vi "TEST Config.vi"() -> ()   [LabVIEW 2013, in "Carya Config.lvclass"]
doc: "Copyright 2018, Carya Automatisering, Wiebe Walstra."
uses:
  Carya Config.lvclass
  CConfig Object/Data.ctl
  CConfig Object/CConfig Object.lvclass
  CConfig Object/Set Query/Set Query.lvclass
  CConfig Object/Step In Query/Step In Query.lvclass
  CConfig Object/Loop Query/Match Query/Match Query.lvclass
  CConfig Object/Loop Query/All Query/All Query.lvclass
panel:
  out "Section names 5":string[](array[string])
  out "Array 2":string[](array[string])
  out "String 7":string
  out "String 6":string
  out "Section names 4":string[](array[string])
  out "Key names 3":string[](array[string])
  out "Key names 2":string[](array[string])
  out "Section names 3":string[](array[string])
  out "Section names 2":string[](array[string])
  out "String 5":string
  out "Key names":string[](array[string])
  out "Section names":string[](array[string])
  out "String 4":string
  out "Section names":string[](array[string])
  out "Key context":string[](array[string])
  out "Key names":string[](array[string])
  out "Section names":string[](array[string])
  out "Array":bool[][](array[boolean])
  out "String 3":string
  out "Found?":bool
  in  "String 2":string="[123]\none=test\na=aval\nb=bval\nc=cval\nd=dval\n13=abcval\n\n[456]\ntwo=abc\nstring=\"\"\nstring2=\"\""
  out "Value":string
  out "String":string
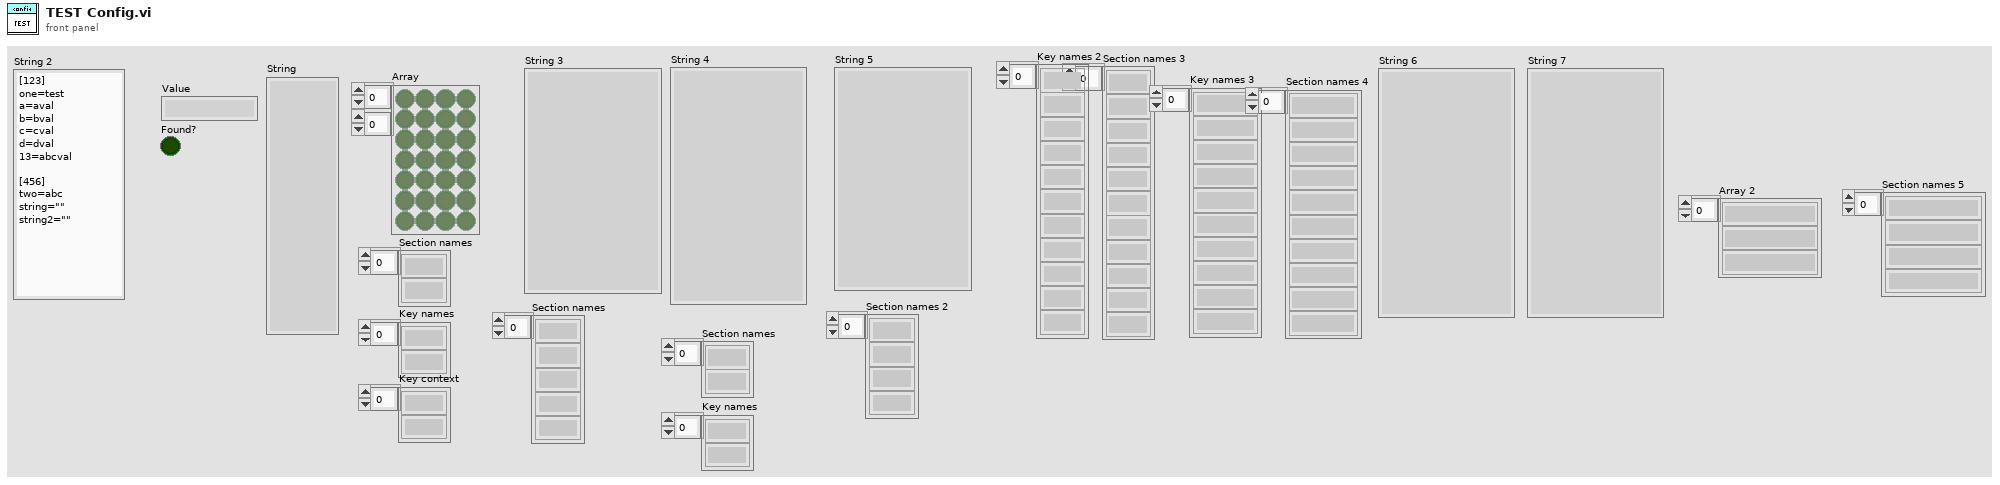
[diagram p1: front panel]
types:
  T1 = typedef "CConfig Object.lvclass/Data.ctl" = enum16{"pre", "name", "middle", "value", "post", "newline", "persistant", "tagged", "type"}
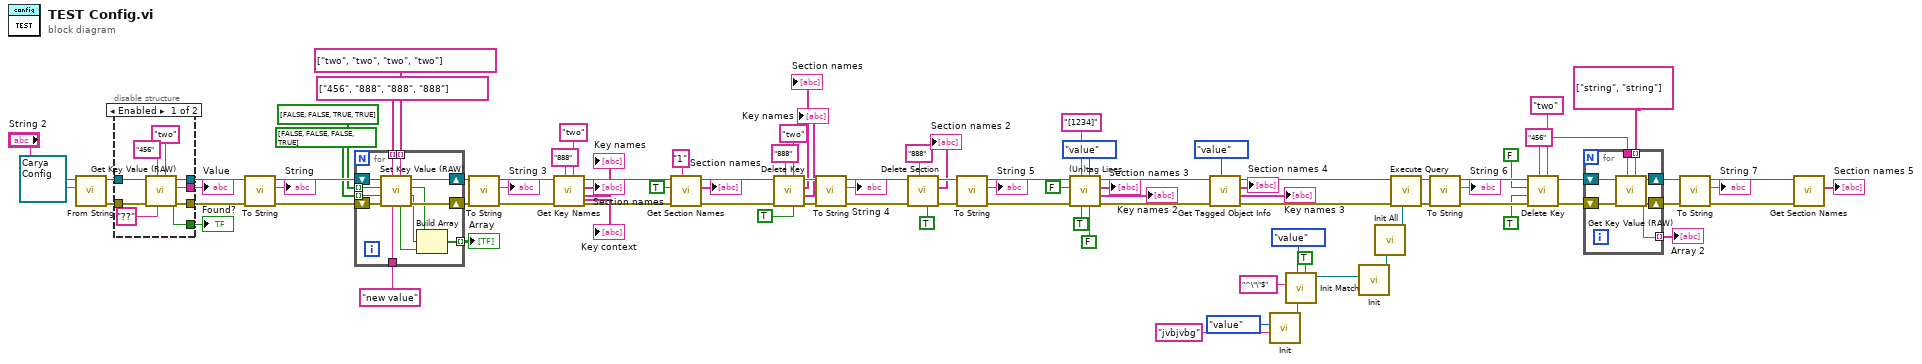
[diagram p0: block diagram]
diagram:
  w8 = "456" ("Section name")
  n1 = call-dynamic "From String.vi"("String"="String 2", "Carya Config in"=refnum<class "Carya Config.lvclass"> refnum) -> ("error out"=w58:errorcluster, "Carya Config out"=w91:refnum<class "Carya Config.lvclass">)  [unwired: 7 in, 1 out]
  n2 = disable-structure shown="Enabled" {
    disable-tunnel: w91 -> [w103 w105]
    disable-tunnel: [w102 w105] -> w90
    disable-tunnel: [w99 _] -> w89
    disable-tunnel: [w98 _] -> w88
    disable-tunnel: [w96 w104] -> w59
    disable-tunnel: w58 -> [w95 w104]
    frame Enabled {
      n3 = call-dynamic "Get Key Value (RAW).vi"("Key name"="two", "Default"="??", "Section name"="456", "error in (no error)"=w95, "Carya Config in"=w103) -> ("error out"=w96:errorcluster, "Found?"=w98:bool, "Value"=w99:string, "Carya Config out"=w102:refnum<class "Carya Config.lvclass">)  [unwired: 3 in]
    }
    frame Disabled {
    }
  }
  "Value" <- w89
  "Found?" <- w88
  n4 = call-dynamic "To String.vi"("error in (no error)"=w59, "Carya Config in"=w90) -> ("error out"=w86:errorcluster, "String"=→"String":string, "Carya Config out"=w87:refnum<class "Carya Config.lvclass">)  [unwired: 7 in]
  n5 = for {
    tunnel: string[] ["456", "888", "888", "888"] -> [w117] mode=indexing
    tunnel: string[] ["two", "two", "two", "two"] -> [w116] mode=indexing
    tunnel: "new value" ("Key value") -> [w114]
    shift-right: [w113] -> w84
    shift-left: w87 -> [w118]
    shift-right: [w112] -> w83
    shift-left: w86 -> [w115]
    tunnel: [w108] -> w79 mode=indexing
    tunnel: bool[] [FALSE, FALSE, TRUE, TRUE] -> [w107] mode=indexing
    tunnel: bool[] [FALSE, FALSE, FALSE, TRUE] -> [w106] mode=indexing
    n6 = call-dynamic "Set Key Value (RAW).vi"("Key name"=w116, "Key value"=w114, "Section name"=w117, "error in (no error)"=w115, "Create key? [T]"=w106, "Create section? [T]"=w107, "Carya Config in"=w118) -> ("error out"=w112:errorcluster, "Created key?"=w110:bool, "Created session?"=w111:bool, "Carya Config out"=w113:refnum<class "Carya Config.lvclass">, "Value written?"=w109:bool)
    n7 = Build Array(w111, w110, w109) -> (w108:bool[])
  }
  "Array" <- w79
  n8 = call-dynamic "To String.vi"("error in (no error)"=w83, "Carya Config in"=w84) -> ("error out"=w77:errorcluster, "String"=→"String 3":string, "Carya Config out"=w47:refnum<class "Carya Config.lvclass">)  [unwired: 7 in]
  n9 = call-dynamic "Get Key Names.vi"("Key name/Regex"="two", "Section name/Regex"="888", "error in (no error)"=w77, "Carya Config in"=w47) -> ("error out"=w70:errorcluster, "Key names"=→"Key names":string[], "Section names"=→"Section names":string[], "Carya Config out"=w71:refnum<class "Carya Config.lvclass">, "Context (concatenated)"=→"Key context":string[])  [unwired: 3 in]
  n10 = call-dynamic "Get Section Names.vi"("Section Regex [\"\", all]"="1" ("Section Regex [\"\", all]"), "error in (no error)"=w70, "Use Regex? [T]"=TRUE, "Carya Config in"=w71) -> ("error out"=w66:errorcluster, "Section names"=→"Section names":string[], "Carya Config out"=w65:refnum<class "Carya Config.lvclass">)  [unwired: 5 in]
  n11 = call-dynamic "Delete Key.vi"("Return deleted names? [F]"=TRUE, "Key name"="two", "Section name"="888", "error in (no error)"=w66, "Carya Config in"=w65) -> ("error out"=w63:errorcluster, "Key names"=→"Key names":string[], "Section names"=→"Section names":string[], "Carya Config out"=w62:refnum<class "Carya Config.lvclass">)  [unwired: 3 in]
  n12 = call-dynamic "To String.vi"("error in (no error)"=w63, "Carya Config in"=w62) -> ("error out"=w53:errorcluster, "String"=→"String 4":string, "Carya Config out"=w54:refnum<class "Carya Config.lvclass">)  [unwired: 7 in]
  n13 = call-dynamic "Delete Section.vi"("Return deleted section names? [F]"=TRUE, "Section name"="888", "error in (no error)"=w53, "Carya Config in"=w54) -> ("error out"=w49:errorcluster, "Section names"=→"Section names 2":string[], "Carya Config out"=w50:refnum<class "Carya Config.lvclass">)  [unwired: 5 in]
  n14 = call-dynamic "To String.vi"("error in (no error)"=w49, "Carya Config in"=w50) -> ("error out"=w45:errorcluster, "String"=→"String 5":string, "Carya Config out"=w46:refnum<class "Carya Config.lvclass">)  [unwired: 7 in]
  n15 = call-dynamic "(Un)tag Lines.vi"("Set if match (T)\\Set it no match (F) [T]"=FALSE ("Set if match (T)\\Set it no match (F) [T]"), "Context [name]"=Data."value" ("Context [Name]"), "Tag (T)\\Untag (F) [T]"=TRUE ("Tag (T)\\Untag (F) [T]"), "String\\Regex [\"\"]"="[1234]" ("String\\Regex [\"\"]"), "error in (no error)"=w45, "Use Regex? [T]"=FALSE, "Carya Config in"=w46) -> ("error out"=w39:errorcluster, "context"=→"Key names 2":string[], "Section names"=→"Section names 3":string[], "Carya Config out"=w40:refnum<class "Carya Config.lvclass">)  [unwired: 1 in]
  n16 = call-dynamic "Get Tagged Object Info.vi"("Context [name]"=Data."value", "error in (no error)"=w39, "Carya Config in"=w40) -> ("error out"=w34:errorcluster, "Context"=→"Key names 3":string[], "Section names"=→"Section names 4":string[], "Carya Config out"=w33:refnum<class "Carya Config.lvclass">)  [unwired: 5 in]
  n17 = call "Init.vi"("Value"="jvbjvbg", "Data [value]"=Data."value" ("Data")) -> ("Set Query out"=w21:refnum<class "Set Query.lvclass">)  [unwired: 8 in, 1 out]
  n18 = call "Init Match.vi"("Regex [F]"=TRUE, "Found"=w21, "Data [name]"=Data."value", "Data"="^\"\"$" ("String\\Regex [\"\"]")) -> ("Find First Query out"=w20:refnum<class "Loop Query.lvclass">)  [unwired: 6 in, 1 out]
  n19 = call "Init.vi"("Config Query"=w20) -> ("Step In Query out"=w22:refnum<class "Step In Query.lvclass">)  [unwired: 9 in, 1 out]
  n20 = call "Init All.vi"("Found"=w22) -> ("Find First Query out"=w19:refnum<class "All Query.lvclass">)  [unwired: 9 in, 1 out]
  n21 = call-dynamic "Execute Query.vi"("Config Query in"=w19, "error in (no error)"=w34, "Carya Config in"=w33) -> ("error out"=w23:errorcluster, "Carya Config out"=w29:refnum<class "Carya Config.lvclass">)  [unwired: 4 in, 3 out]
  n22 = call-dynamic "To String.vi"("error in (no error)"=w23, "Carya Config in"=w29) -> ("error out"=w17:errorcluster, "String"=→"String 6":string, "Carya Config out"=w15:refnum<class "Carya Config.lvclass">)  [unwired: 7 in]
  n23 = call-dynamic "Delete Key.vi"("Key name"="two", "Section name"=w8, "error in (no error)"=w17, "Use Key Regex? [F]"=TRUE, "Use Section Regex? [F]"=FALSE, "Carya Config in"=w15) -> ("error out"=w16:errorcluster, "Carya Config out"=w10:refnum<class "Carya Config.lvclass">)  [unwired: 2 in, 2 out]
  n24 = for {
    tunnel: w8 -> [w121]
    shift-right: [w122] -> w9
    shift-left: w10 -> [w123]
    shift-right: [w124] -> w11
    shift-left: w16 -> [w125]
    tunnel: string[] ["string", "string"] -> [w120] mode=indexing
    tunnel: [w119] -> w6 mode=indexing
    n25 = call-dynamic "Get Key Value (RAW).vi"("Key name"=w120, "Section name"=w121, "error in (no error)"=w125, "Carya Config in"=w123) -> ("error out"=w124:errorcluster, "Value"=w119:string, "Carya Config out"=w122:refnum<class "Carya Config.lvclass">)  [unwired: 4 in, 1 out]
  }
  "Array 2" <- w6
  n26 = call-dynamic "To String.vi"("error in (no error)"=w11, "Carya Config in"=w9) -> ("error out"=w4:errorcluster, "String"=→"String 7":string, "Carya Config out"=w5:refnum<class "Carya Config.lvclass">)  [unwired: 7 in]
  n27 = call-dynamic "Get Section Names.vi"("error in (no error)"=w4, "Carya Config in"=w5) -> ("Section names"=→"Section names 5":string[])  [unwired: 7 in, 2 out]
